vi "LWXPS_ErrorStringGet.vi"(0 "XPS Reference IN":refnum<k24>, 5 "ErrorCode":i32, 11 "LabVIEW error IN":errorcluster) -> (4 "XPS Reference OUT":refnum<k24>, 6 "Error String":string, 8 "Returned error code":i32, 10 "XPS Error String":string, 15 "LabVIEW error OUT":errorcluster)   [LabVIEW 2014]
uses:
  D:/XPSQ8_LabView_Library/Development/Source/Dll/Newport.XPS.CommandInterface.dll
  Dll/Newport.XPS.CommandInterface.dll
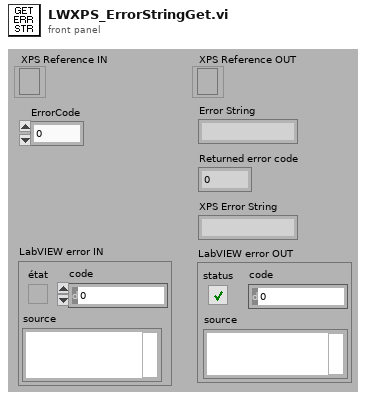
[diagram p1: front panel]
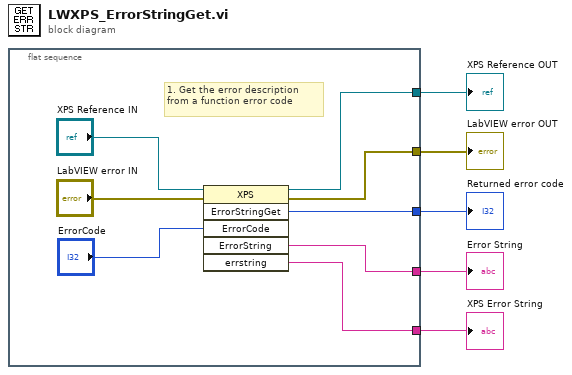
[diagram p0: block diagram]
diagram:
  n1 = flat-sequence {
    tunnel: [w10] -> w5
    tunnel: [w13] -> w4
    tunnel: [w9] -> w1
    tunnel: [w6] -> w3
    tunnel: [w8] -> w2
    frame #0 {
      # "1. Get the error description from a function error code"
      n2 = invoke class="XPS" method="ErrorStringGet"(reference="XPS Reference IN", error in="LabVIEW error IN", "ErrorCode"="ErrorCode") -> (reference out=w10:refnum<k24>, error out=w13:errorcluster, "ErrorStringGet"=w9:i32, "ErrorString"=w6:string, "errstring"=w8:string)  [unwired: 3 in, 1 out]
    }
  }
  "XPS Reference OUT" <- w5
  "LabVIEW error OUT" <- w4
  "Error String" <- w3
  "XPS Error String" <- w2
  "Returned error code" <- w1
